vi "AppClose.vi"(8 "error in (no error)":errorcluster) -> ()   [LabVIEW 2016]
uses:
  Global/ApplicationGlobal.vi
  tools/Translator/Translator.Message.ctl
  tools/Translator/Translator.Control.Fglb.Action.vi
  tools/EventLog/EventLog.New(single).vi
  tools/EventLog/EventLog.Buffer.Action.ctl
  tools/Translator/Translator.Global.vi
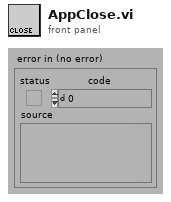
[diagram p1: front panel]
types:
  T1 = typedef "Translator.Control.Fglb.Action.vi" = enum16{"init", "set", "get", "clear"}
  T2 = typedef "Translator.Message.ctl" = enum16{"-", "Event confirmed", "Log out", "Log in", "Shutdown", "Cancel", "Start", "Begin time", "End time", "Duration", "Service Mode", "Ignore Results", "Serial Format", "On", "Off", "OK", "NOK", "NOK %s", "Home", "Work", "Close", "Open", "In progress...", "Missing", "Empty", "Hardware failure", "Initial", "Default", "Total", "Out of range", "Free disk space is below 1GB - contact technician", "Error %d >> %s", "Error %d >> %s >> %s", "Msg %d >> %s", "Laser msg %d %s", "Laser cmd error %s %d", "Laser cmd failed %s", "Laser cmd warning %s", "Laser disconnected", "Laser status %s", "Laser already started", "Laser job unkonwn %s", "Laser job missing %s", "Laser job select failure %s", "Unable to start laser printing (%s)", "Unable to stop laser printing (%s)", "Laser marking aborted", "Laser marking timeout", "Unable to reset Laser Interlock (%s)", "Unable to trigger Laser. Laser not ready (%s)", "Laser job '%s' coordinates not configured", "Starting %s", "Quitting %s", "Configured", "Initializing", "Quitting", "Loading", "Loaded %d results", "Loaded %d events", "Running", "Stopped", "Summary", "Laser", "Do you want to continue?", "Do you want to delete the configuration?", "The configuration is being used by an order. Unable to delete!", "Press confirm button", "Station is not based. Do you want to exit?", "Station requires changeover. Do you want to run the test?", "Test options are not set as default. Do you want to continue?", "Formatting of WabcoNo is disabled. Do you want to continue?", "Product not detected. Do you want to continue?", "Product scan failed. Do you want to continue?", "Calibration", "Log out?", "System", "All", "IDLE", "Translating...%s", "Not found", "Alarm %s", "Run", "Skip", "Abort", "Repeat", "Please wait...", "Database disconnected", "Database disconnected - changeover disabled!", "Login to database successful", "Login to database failed: %d; %s", "Unable to check the product status of reference %d - database disconnected", "Unable to set the product status of reference %d - database disconnected", "Variant file backup %s", "Read variant (%s)", "Result", "Station armed!", "Station requires changeover!", "Select reference number...", "EMERGENCY BUTTON - press Control button", "EMERGENCY DOOR - press Control button", "Resetting Emergency...", "Unable to reset safety circuit - Emergency Button pressed", "Unable to reset safety circuit - Emergency Side Door open", "Station not based", "Station based", "Station not empty", "Station basing...", "No order", "Press Start to begin new order", "Scanning new order", "Order NOK. Correct or scan again", "Order OK. Press Accept", "Order ready", "Revolver incorrect", "Fork incorrect", "Revolver missing", "Revolver empty", "Container missing", "Offline results", "Offline statistics", "Updating statistics %.1f %%", "DMC Configurator", "Door open", "Close the front door", "Press start button", "Done. Open the front door", "Running...", "Running...%.1f %%", "Pause %s", "Pause %s. NOK container missing", "Pause %s. OK container missing", "Pause %s. Revolver empty", "Pause %s. Revolver missing", "Pause %s. Revolver incorrect", "Pause %s. Fork missing", "Pause %s. Fork incorrect", "Pause %s. Too many failures", "Pause %s. Unloading failure", "Pause %s. One slot is not working", "Pause %s. Part order is done. Empty OK container", "Pause %s. Unable to move product to slot", "Pause %s. Unable to move back product pusher", "Pause %s. Unable to lift product", "Pause %s. Unable to move back product lifter", "Pause %s. Unable to move product arm to Work", "Pause %s. Unable to move product arm to NOK", "Pause %s. Unable to move product arm to OK", "Pause %s. Unable to unsuck the NOK product", "Pause %s. Unable to drop the NOK product", "Pause %s. Product OK missing", "Pause %s. Unable to unsuck the OK product", "Pause %s. Unable to drop the OK product", "Stopping...", "File '%s' is missing", "File '%s' is broken", "File '%s' is running", "Log file started (%s)", "Log file ended (%s)", "Log file stopped (%s)", "Log file ignored (%s)", "Log file exported (%s)", "Log file export failed (%s)", "Wrong serial number in log file", "Wrong reference number in log file", "Test steps are missing", "%s = %.3f", "Process param '%s' not found in DB", "Process param '%s' wrong order", "Process param '%s' value %.3f out of limits (%.3f; %.3f)", "Step%d param '%s' not found in DB", "Step%d param '%s' wrong order", "Step%d param '%s' value %.3f out of limits (%.3f; %.3f)", "Step%d EV '%s' not found in DB", "Step%d EV '%s' wrong order", "\"%s\" not found in DB", "\"%s\" wrong order", "\"%s\" value %.3f out of limits (%.3f; %.3f)", "\"%s\" not found in software", "Process init (%s)", "Process started", "Process restarted", "Process run", "Process done", "Process done - remove OK container", "Process aborted", "Process aborted at work", "Process aborted at home", "Process error", "Process error at home", "Process error at work", "Process close", "Process pause", "Process continue", "Process door open", "Process door close", "Process pause at slot %s due to %s", "Select plate from the order to process", "Do you want to start the process?", "Do you want to continue the process?", "There is unfinished order. Do you want to put the new order?", "Product %s %d OK", "Product %s %d NOK", "Unable to unload the slot %s. Product missing in the slot", "Unable to unload the slot %s. Product already in the arm", "Unable to accept the product as OK. Product missing in slot %s", "Unable to accept the product as OK. Product could not drop into the container at slot %s", "Unable to accept the product as NOK. Product could not drop into the container at slot %s", "Scan failed. Error %s", "Scan failed. Scanner disconnected", "Scan failed. Wrong Wabco number %d, limit (%d,%d)", "Scan failed. Wrong serial number %d, limit (%d,%d)", "Scan failed. Wrong date %d, limit (%d,%d)", "Scan failed. Wrong product wabco number %d (expected %d)", "Scan failed. Wrong product serial number %d (expected > 0)", "Scan OK %s", "Scan failed. Unable to determine table position (%s)", "Scan failed. Timeout", "Tune failed. Scanner disconnected", "Tune failed. Timeout", "%s = %d", "%s = %d->%d", "Unable to set %s = %.2f - Air Pressure Inside off", "Unable to set digital output '%s' = %d", "Unable to activate air pressure inside - timeout", "Unable to activate air pressure inside - aborted", "Unable to switch on Air Main Valve - Air Pressure Inlet off", "Unable to switch on Air Main Valve - Door open", "Unable to switch off Air Main Valve - timeout", "Unable to switch off Air Main Valve - aborted", "Unable to rotate Table - timeout", "Unable to rotate Table - aborted", "Unable to rotate Table - Product Move not in Home position", "Unable to rotate Table - Air Pressure Inside off", "Unable to rotate Table - Product Lift A not in Home position", "Unable to rotate Table - Product Lift B not in Home position", "Unable to rotate Table - unlock before movement timeout", "Unable to rotate Table - lock after movement timeout", "Unable to move Table Lock to %s position - timeout", "Unable to move Table Lock to %s position - aborted", "Unable to move Table Lock to %s position - Air Pressure Inside off", "Unable to move Table Lock to %s position - Table not in position", "Unable to move Product Lift A to %s position - timeout", "Unable to move Product Lift B to %s position - timeout", "Unable to move Product Lift A to %s position - aborted", "Unable to move Product Lift B to %s position - aborted", "Unable to move Product Lift A to %s position - Air Pressure Inside off", "Unable to move Product Lift B to %s position - Air Pressure Inside off", "Unable to move Product Lift A to %s position - Table not locked", "Unable to move Product Lift B to %s position - Table not locked", "Unable to move Product Lift A to %s position - Product Arm not in Work position", "Unable to move Product Lift B to %s position - Product Arm not in Work position", "Unable to set Product Suction Gripper %s to %s - timeout", "Unable to set Product Suction Gripper %s to %s - aborted", "Unable to set Product Suction Gripper %s to %s - Air Pressure Inside off", "Unable to set Product Suction Gripper %s to %s - Table slot unkown", "Unable to move Product Arm to %s position - timeout", "Unable to move Product Arm to %s position - aborted", "Unable to move Product Arm to %s position - Air Pressure Inside off", "Unable to move Product Arm to %s position - Product Lift A not in Home position", "Unable to move Product Arm to %s position - Product Lift B not in Home position", "Unable to move Product to %s position - timeout", "Unable to move Product to %s position - aborted", "Unable to move Product to %s position - Air Pressure Inside off", "Unable to move Product to %s position - Table not in position"}
  T3 = enum32{"Invalid", "Standard", "Closed", "Hidden", "Minimized", "Maximized"}
  T4 = typedef "EventLog.Buffer.Action.ctl" = enum16{"init", "re-init", "clear", "set translator", "add", "get", "get unsaved"}
  T5 = typedef "EventLog.EventGui.ctl" = cluster{"ts":dbl, "lev":T6, "usr":i32, "src":T7, "msg":T2, "arg":variant[], "msg_str":string}
  T6 = typedef "EventLog.EventLevel.ctl" = enum8{"Debug", "Info", "Warning", "Error"}
  T7 = typedef "EventLog.EventSource.ctl" = enum16{"All", "Gui", "Ref", "File", "Arch", "Seq", "CPX", "DB", "Laser", "Scan.P", "Scan.O"}
  T8 = cluster{"ts":dbl, "lev":T6, "usr":i32, "src":T7, "msg":T2, "arg":variant[]}
  T9 = typedef "Windows.ExitAction.ctl" = enum16{"Log off from PC", "Shut Down PC", "Reboot PC", "Close Program"}
  T10 = enum32{"invalid app kind", "Development System", "Run Time System", "Student Edition", "Embedded LabVIEW", "Evaluation", "Custom"}
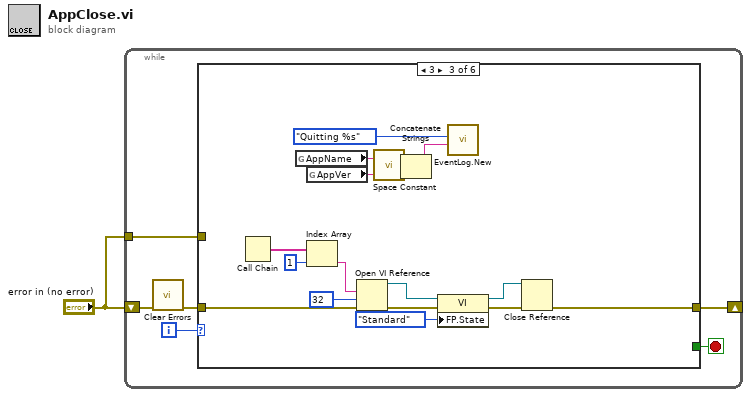
[diagram p0: block diagram]
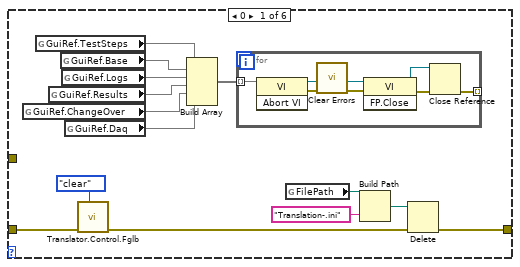
[diagram p2: hidden frame]
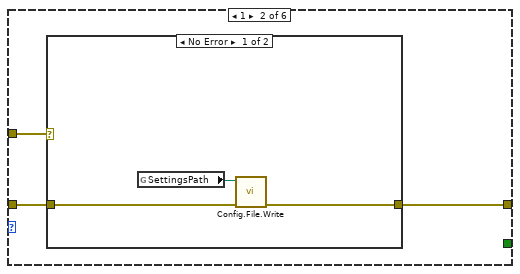
[diagram p3: hidden frame]
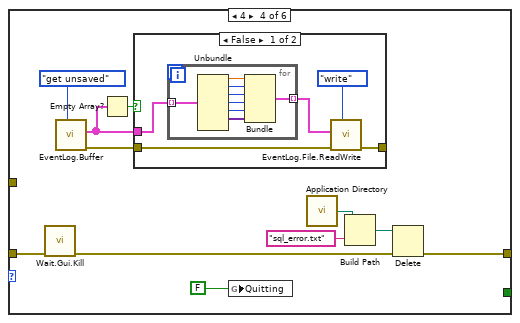
[diagram p5: hidden frame]
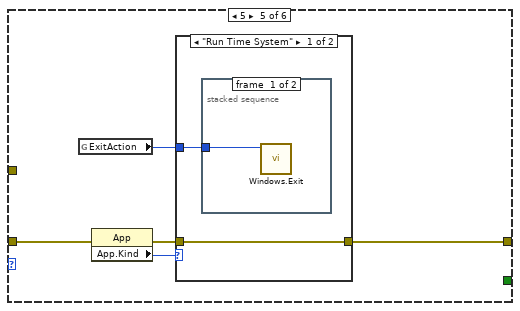
[diagram p7: hidden frame]
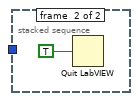
[diagram p8: hidden frame]
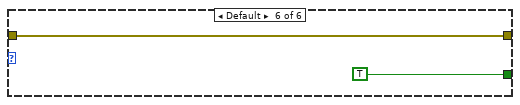
[diagram p10: hidden frame]
diagram:
  n1 = while {
    shift-right: [w3] -> _
    shift-left: "error in (no error)" -> [w5]
    tunnel: "error in (no error)" -> [w2]
    i -> [w7]
    stop <- w6 stop-if-true
    n2 = call <vilib>:"Clear Errors.vi"("error in (no error)"=w5) -> ("error out"=w4:errorcluster)  [unwired: 5 in, 1 out]
    n3 = case shown="3" w7 {
      tunnel: [_ _ _ _ _ TRUE] -> w6
      tunnel: w4 -> [w20 w30 w43 w62 w78 w87]
      tunnel: [w8 w31 w42 w53 w77 w87] -> w3
      tunnel: w2 -> [_ w29 _ _ _ _]
      frame 0 {
        n4 = global read "ApplicationGlobal.vi" "GuiRef.ChangeOver"() -> (w15)
        n5 = global read "ApplicationGlobal.vi" "GuiRef.TestSteps"() -> (w19)
        n6 = global read "ApplicationGlobal.vi" "GuiRef.Results"() -> (w16)
        n7 = global read "ApplicationGlobal.vi" "GuiRef.Base"() -> (w18)
        n8 = global read "ApplicationGlobal.vi" "GuiRef.Logs"() -> (w17)
        n9 = global read "ApplicationGlobal.vi" "GuiRef.Daq"() -> (w14)
        n10 = call "Translator.Control.Fglb.vi"("Action"=Translator.Control.Fglb.Action.vi."clear", "error in (no error)"=w20) -> ("error out"=w9:errorcluster)  [unwired: 8 in, 1 out]
        n11 = Build Array(w19, w18, w17, w16, w15, w14) -> (w13:void[])
        n12 = for {
          tunnel: w13 -> [w25] mode=indexing
          tunnel: [w26] -> _ mode=indexing
          n13 = invoke class="VI" method="Abort VI"(reference=w25) -> (reference out=w24:refnum<vi>, error out=w23:errorcluster)  [unwired: 2 in, 1 out]
          n14 = call <vilib>:"Clear Errors.vi"("error in (no error)"=w23) -> ("error out"=w22:errorcluster)  [unwired: 5 in, 1 out]
          n15 = invoke class="VI" method="FP.Close"(reference=w24, error in=w22) -> (reference out=w28:refnum<vi>, error out=w27:errorcluster)  [unwired: 1 in, 1 out]
          n16 = Close Reference(reference=w28, error in (no error)=w27) -> (error out=w26:errorcluster)
        }
        n17 = global read "Translator.Global.vi" "FilePath"() -> (w11:path)
        n18 = Build Path(base path=w11, name or relative path="Translation-.ini") -> (appended path=w10:path)
        n19 = Delete(path (use dialog)=w10, error in=w9) -> (error out=w8:errorcluster)  [unwired: 3 in, 2 out]
      }
      frame 1 {
        n20 = case shown="No Error" w29 {
          tunnel: [w34 w35] -> w31
          tunnel: w30 -> [w33 w35]
          frame No Error {
            n21 = global read "ApplicationGlobal.vi" "SettingsPath"() -> (w32:path)
            n22 = call "Config.File.Write.vi"("error in"=w33, "path"=w32) -> ("error out"=w34:errorcluster)  [unwired: 9 in]
          }
          frame Error {
          }
        }
      }
      frame 3 {
        n23 = Call Chain() -> (call chain=w46:string[])
        n24 = global read "ApplicationGlobal.vi" "AppName"() -> (w40:string)
        n25 = global read "ApplicationGlobal.vi" "AppVer"() -> (w39:string)
        n26 = Index Array(array=w46, index=1) -> (element=w44:string)
        n27 = Open VI Reference(vi path=w44, options=32, error in (no error)=w43) -> (vi reference=w49:refnum<vi>, error out=w50:errorcluster)  [unwired: 3 in]
        n28 = call <vilib>:"Space Constant.vi"() -> ("String"=w38:string)
        n29 = Concatenate Strings(w40, w38, w39) -> (w37:string)
        n30 = property class="VI"(reference=w49, error in=w50, "FP.State"=T3."Standard" ("Front Panel Window:State")) -> (reference out=w47:refnum<vi>, error out=w48:errorcluster)
        n31 = call-poly "EventLog.New.vi"("Arg"=w37, "Message (-)"=Translator.Message."Quitting %s") -> ()  [unwired: 8 in, 2 out]
        n32 = Close Reference(reference=w47, error in (no error)=w48) -> (error out=w42:errorcluster)
      }
      frame 4 {
        n33 = call "Wait.Gui.Kill.vi"("error in (no error)"=w62) -> ("error out"=w54:errorcluster)  [unwired: 10 in]
        n34 = call "EventLog.Buffer.vi"("action (get)"=EventLog.Buffer.Action."get unsaved") -> ("error out"=w59:errorcluster, "data out"=w58:T5[])  [unwired: 7 in, 2 out]
        n35 = Empty Array?(array=w58) -> (empty?=w57:bool)
        n36 = case shown="False" w57 {
          tunnel: w59 -> [w66 w76]
          tunnel: w58 -> [w64 _]
          tunnel: [w65 w76] -> _
          frame False {
            n37 = for {
              tunnel: w64 -> [w75] mode=indexing
              tunnel: [w68] -> w63 mode=indexing
              n38 = Unbundle(w75) -> ("ts"=w74:dbl, "lev"=w73:T6, "usr"=w71:i32, "src"=w72:T7, "msg"=w70:T2, "arg"=w69:variant[])  [unwired: 1 out]
              n39 = Bundle("ts"=w74, "lev"=w73, "usr"=w71, "src"=w72, "msg"=w70, "arg"=w69) -> (w68:T8)  [unwired: 1 in]
            }
            n40 = call "EventLog.File.ReadWrite.vi"("action (read)"=enum16{"read", "write"}."write", "error in"=w66, "Events in"=w63) -> ("error out"=w65:errorcluster)  [unwired: 4 in, 4 out]
          }
          frame True {
          }
        }
        n41 = global write "ApplicationGlobal.vi" "Quitting"(FALSE ("Quitting")) -> ()
        n42 = call <vilib>:"Application Directory.vi"() -> ("Application Directory"=w52:path)
        n43 = Build Path(base path=w52, name or relative path="sql_error.txt") -> (appended path=w55:path)
        n44 = Delete(path (use dialog)=w55, error in=w54) -> (error out=w53:errorcluster)  [unwired: 3 in, 2 out]
      }
      frame 5 {
        n45 = global read "ApplicationGlobal.vi" "ExitAction"() -> (w79:T9)
        n46 = property class="App"(error in=w78) -> (error out=w80:errorcluster, "App.Kind"=w81:T10)  [unwired: 1 in, 1 out]
        n47 = case shown="\"Run Time System\"" w81 {
          tunnel: w80 -> [w82 w86]
          tunnel: w79 -> [w83 _]
          tunnel: [w82 w86] -> w77
          frame "Run Time System" {
            n48 = stacked-sequence {
              tunnel: w83 -> [w84 _]
              frame #0 {
                n49 = call "Windows.Exit.vi"("Exit Action"=w84) -> ()  [unwired: 6 in, 1 out]
              }
              frame #1 {
                n50 = Quit LabVIEW(quit? (T)=TRUE) -> ()
              }
            }
          }
          frame Default {
          }
        }
      }
      frame Default {
      }
    }
  }
